vi "Get_EXE_Path.vi"(11 "Installer in":refnum<class "Installer.lvclass">) -> (0 "run?":bool, 1 "cmdArg":string, 2 "exe path":string, 3 "Installer out":refnum<class "Installer.lvclass">)   [LabVIEW 2020, in "Installer.lvclass"]
uses:
  <vilib>/AppBuilder/IB_Classes/Installer/Installer.lvclass
  <vilib>/AppBuilder/IB_Classes/Installer/Installer.lvclass/Installer.ctl
  <vilib>/AppBuilder/IB_Classes/Source/File/IB_Source_File.lvclass
  <vilib>/AppBuilder/IB_Classes/Source/IB_Source.lvclass
  e:/builds/penguin/labview/branches/2020/dev/dist/vi.lib/AppBuilder/IB_Classes/Source/IB_Source.lvclass
  e:/builds/penguin/labview/branches/2020/dev/dist/vi.lib/AppBuilder/IB_Classes/Source/File/IB_Source_File.lvclass
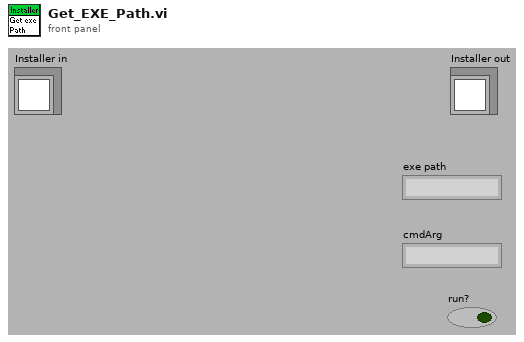
[diagram p1: front panel]
types:
  T1 = typedef "IB_Installer.ctl" = cluster{"Destination":refnum<class "IB_Destination.lvclass">[], "Source":refnum<class "IB_Source.lvclass">[], "buildObject":T2, "defaultDir":string, "platform":string, "author":string, "productName":string, "buildSpecName":string, "hide":bool, "requireLVDevSys":bool, "autoIncrement":bool, "includeError":bool, "readmeID":string, "buildLocation":path, "readmePath":path, "mediaSize":u16, "language":T3, "productVersion":T4, "preview":bool, "programmatic":bool, "progressBarEvents":T5, "userLog_Path":path, "shortcutAddresses":T7[], "EXE_Install Address":string, "EXE_Uninstall Address":string, "additional NIPaths":refnum<class "Dest_NI_NIPath.lvclass">[], "web service itemIDs":string[], "installerName":string}
  T2 = typedef "ItemRef.ctl" = u64
  T3 = typedef "CDK_sTypeDef_Languages.ctl" = u16
  T4 = typedef "CDK_sTypeDef_ProductVersion.ctl" = cluster{"Major":u8, "Minor":u8, "Update":u16}
  T5 = typedef "provcom_ProgressBar_Events.ctl" = cluster{"newJob":refnum<user-event>, "newItem":refnum<user-event>, "errorMsg":T6, "cancel":refnum<user-event>}
  T6 = typedef "mxLvBuildError.ctl" = refnum<user-event>
  T7 = typedef "CDK_sTypeDef_ShortcutAddress.ctl" = cluster{"file":string, "shortcut":string}
  T8 = typedef "IB_Source_File.ctl" = cluster{"Attributes":i16, "RegCOM":bool, "unlock":bool, "shortcuts":refnum<class "IB_Shortcut.lvclass">[], "EXE_install":bool, "CmdArg_install":string, "EXE_uninstall":bool, "CmdArg_uninstall":string}
  T9 = typedef "IB_Source.ctl" = cluster{"name":string, "sourceTag":string, "destTag":string, "path":path, "eng_installPath":string, "UI_inBuild?":bool, "str ref?":bool}
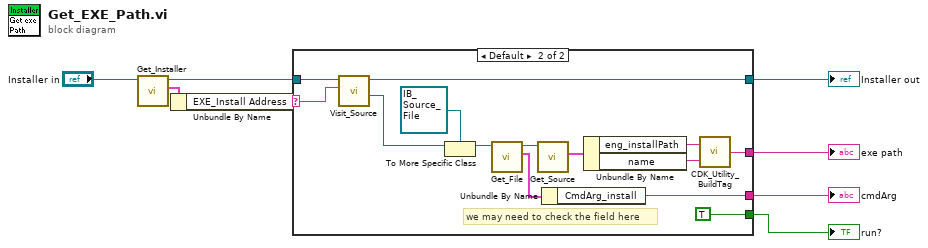
[diagram p0: block diagram]
diagram:
  n1 = call <vilib>:"Get_Installer.vi"("Installer in"="Installer in") -> ("data"=w3:T1, "Installer out"=w5:refnum<class "Installer.lvclass">)  [unwired: 1 in, 8 out]
  n2 = Unbundle By Name(w3) -> ("EXE_Install Address"=w7:string)
  n3 = case shown="Default" w7 {
    selector: w7 -> [_ w11]
    tunnel: [_ w23] -> w1
    tunnel: [_ w22] -> w2
    tunnel: w5 -> [w9 w21]
    tunnel: [w9 w20] -> w6
    tunnel: [_ TRUE] -> w8
    frame "" {
    }
    frame Default {
      # "we may need to check the field here"
      n4 = call <vilib>:"Visit_Source.vi"("address"=w11, "Installer in"=w21) -> ("source"=w10:refnum<class "IB_Source.lvclass">, "Installer out"=w20:refnum<class "Installer.lvclass">)  [unwired: 1 in, 7 out]
      n5 = To More Specific Class(target class=refnum<class "IB_Source_File.lvclass"> refnum ("IB_Source_File.lvclass"), reference=w10) -> (specific class reference=w13:refnum<class "IB_Source_File.lvclass">)  [unwired: 1 in, 1 out]
      n6 = call <vilib>:"Get_File.vi"("IB_Source_File in"=w13) -> ("data"=w16:T8, "IB_Source_File out"=w15:refnum<class "IB_Source_File.lvclass">)  [unwired: 1 in, 8 out]
      n7 = call <vilib>:"Get_Source.vi"("IB_Source in"=w15) -> ("data"=w19:T9)  [unwired: 1 in, 9 out]
      n8 = Unbundle By Name(w16) -> ("CmdArg_install"=w22:string)
      n9 = Unbundle By Name(w19) -> ("eng_installPath"=w18:string, "name"=w17:string)
      n10 = call <resource>:"CDK_Utility_BuildTag.vi"("name or relative path"=w17, "BasePath"=w18) -> ("appended path"=w23:string)
    }
  }
  "run?" <- w8
  "Installer out" <- w6
  "cmdArg" <- w2
  "exe path" <- w1
